vi "Test_RetrievePreviousItem_RetrieveItem.vi"(8 "error in (no error)":errorcluster, 11 "TestCase in":refnum<class "TestStringList.lvclass">) -> (0 "error out":errorcluster, 3 "TestCase out":refnum<class "TestStringList.lvclass">)   [LabVIEW 2015, in "TestStringList.lvclass"]
uses:
  TestStringList.lvclass
  <vilib>/addons/_JKI Toolkits/VI Tester/TestCase.llb/TestCase.lvclass
  StringList.lvclass
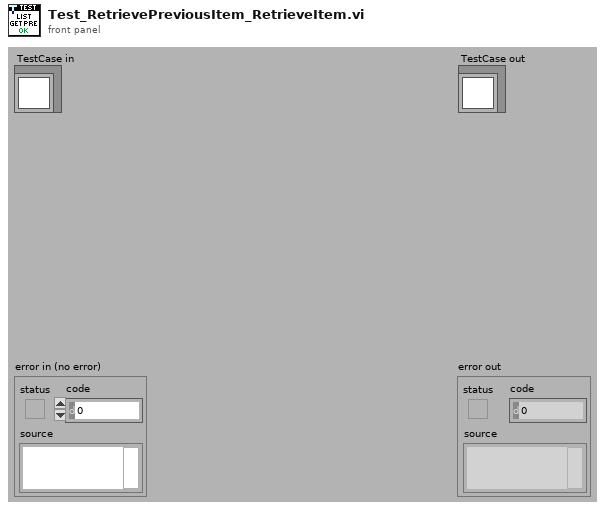
[diagram p1: front panel]
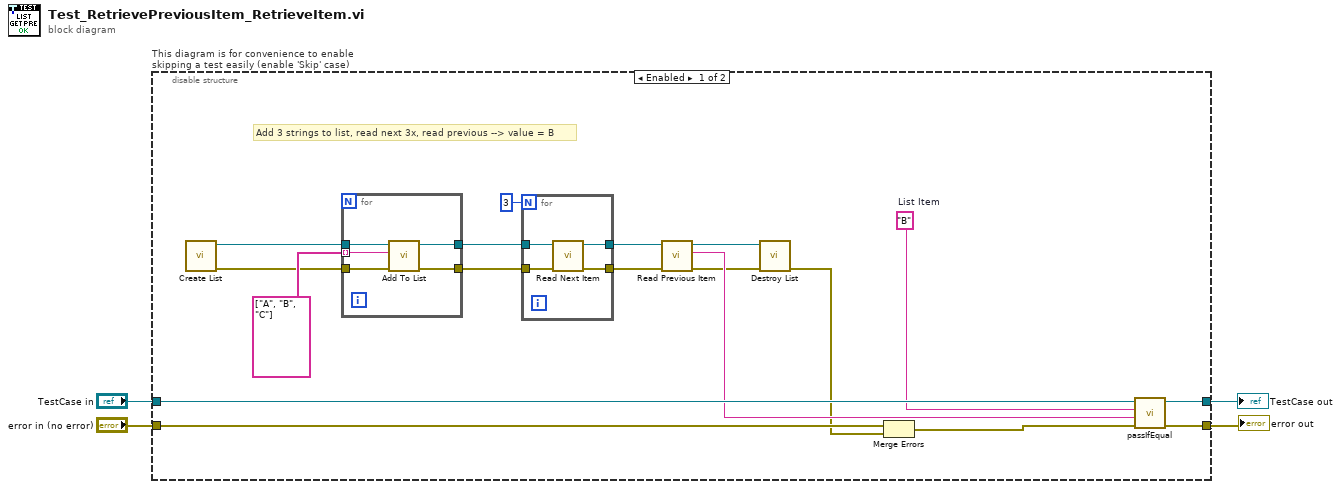
[diagram p0: block diagram]
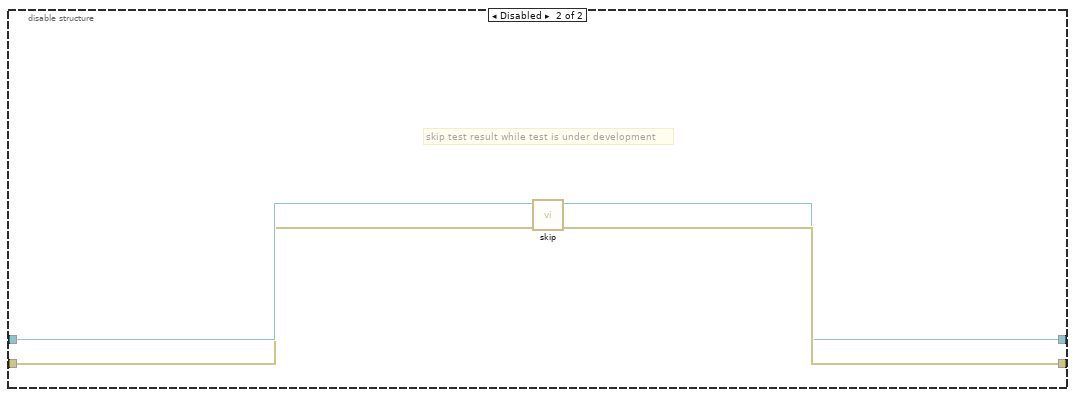
[diagram p2: hidden frame]
diagram:
  n1 = disable-structure "This diagram is for convenience to enable skipping a test easily (enable 'Skip' case)" shown="Enabled" {
    disable-tunnel: "TestCase in" -> [w22 w35]
    disable-tunnel: [w21 w33] -> w1
    disable-tunnel: [w20 w34] -> w3
    disable-tunnel: "error in (no error)" -> [w19 w32]
    frame Enabled {
      w18 = "B"  # List Item
      # "Add 3 strings to list, read next 3x, read previous --> value = B"
      n2 = call "Create List.vi"() -> ("error out"=w11:errorcluster, "StringList Reference"=w12:refnum<data-value>)  [unwired: 10 in]
      n3 = for {
        tunnel: string[] ["A", "B", "C"] -> [w29] mode=indexing
        tunnel: w12 -> [w31]
        tunnel: [w30] -> w17
        tunnel: w11 -> [w28]
        tunnel: [w27] -> w10
        n4 = call "Add To List.vi"("error in (no error)"=w28, "Item"=w29, "StringList Reference"=w31) -> ("error out"=w27:errorcluster, "StringList Reference"=w30:refnum<data-value>)  [unwired: 7 in]
      }
      n5 = for {
        N: 3 -> [_]
        tunnel: w17 -> [w26]
        tunnel: [w25] -> w14
        tunnel: w10 -> [w24]
        tunnel: [w23] -> w9
        n6 = call "Read Next Item.vi"("error in (no error)"=w24, "StringList Reference"=w26) -> ("error out"=w23:errorcluster, "StringList Reference"=w25:refnum<data-value>)  [unwired: 6 in, 2 out]
      }
      n7 = call "Read Previous Item.vi"("error in (no error)"=w9, "StringList Reference"=w14) -> ("error out"=w7:errorcluster, "Item"=w13:string, "StringList Reference"=w8:refnum<data-value>)  [unwired: 6 in, 1 out]
      n8 = call "Destroy List.vi"("error in (no error)"=w7, "StringList Reference"=w8) -> ("error out"=w5:errorcluster)  [unwired: 8 in, 1 out]
      n9 = Merge Errors(w19, w5) -> (w6:errorcluster)
      n10 = call-dynamic "passIfEqual.vi"("error in (no error)"=w6, "y"=w13, "x"=w18, "TestCase in"=w22) -> ("error out"=w20:errorcluster, "TestCase out"=w21:refnum<class "TestStringList.lvclass">)  [unwired: 6 in]
    }
    frame Disabled {
      # "skip test result while test is under development"
      n11 = call <vilib>:"skip.vi"("error in (no error)"=w32, "TestCase in"=w35) -> ("error out"=w34:errorcluster, "TestCase out"=w33:refnum<class "TestStringList.lvclass">)  [unwired: 8 in]
    }
  }
  "error out" <- w3
  "TestCase out" <- w1
